vi "GoblePaths.vi"(8 "error in (no error)":errorcluster caption="错误输入（无错误）", 11 "文件名称":string) -> (0 "error out":errorcluster caption="错误输出", 2 "文件完整路径":path, 3 "文件路径":path)   [LabVIEW 2018]
panel:
  out "文件夹路径":path[](array[path])
  out "文件夹名":string[](array[string])
  out "路径输出":path
  out "Application Directory":path caption="应用程序目录"
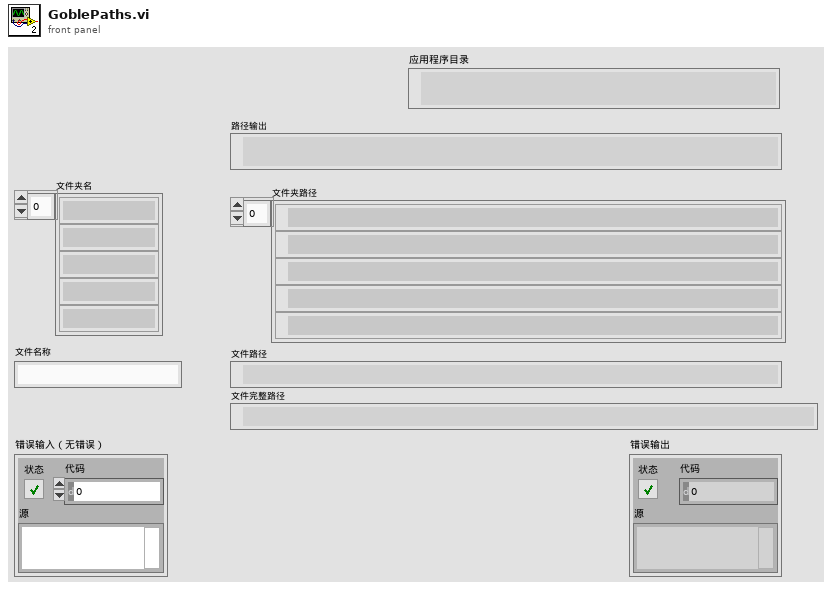
[diagram p1: front panel]
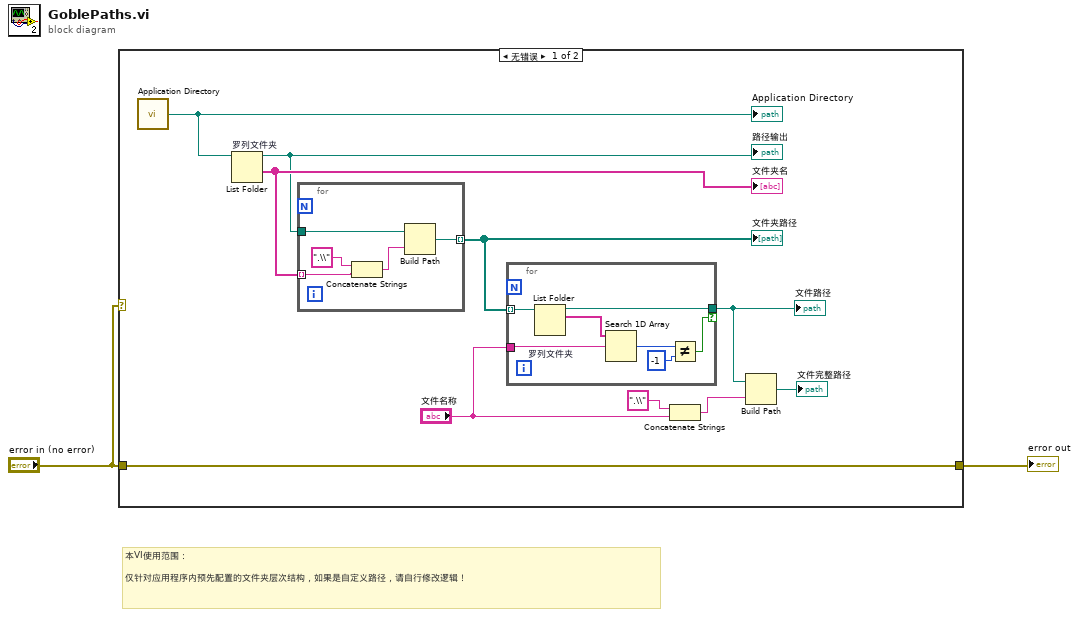
[diagram p0: block diagram]
diagram:
  # "本VI使用范围：\n\n仅针对应用程序内预先配置的文件夹层次结构，如果是自定义路径，请自行修改逻辑！"
  n1 = case shown="无错误" "error in (no error)" {
    tunnel: "error in (no error)" -> [w8 w25]
    tunnel: [w8 w25] -> w2
    frame No Error {
      n2 = call <vilib>:"Application Directory.vi"() -> ("Application Directory"=w12:path)
      "Application Directory" <- w12
      n3 = List Folder "罗列文件夹"(path=w12) -> (path out=w10:path, folder names=w11:string[])  [unwired: 3 in, 2 out]
      "路径输出" <- w10
      "文件夹名" <- w11
      n4 = for {
        tunnel: w11 -> [w22] mode=indexing
        tunnel: w10 -> [w24]
        tunnel: [w20] -> w9 mode=indexing
        n5 = Concatenate Strings(".\\" ("字符串"), w22) -> (w23:string)
        n6 = Build Path(base path=w24, name or relative path=w23) -> (appended path=w20:path)
      }
      "文件夹路径" <- w9
      n7 = for {
        tunnel: w9 -> [w19] mode=indexing
        tunnel: "文件名称" -> [w16]
        tunnel: [w18] -> w7 if=w13
        n8 = List Folder "罗列文件夹"(path=w19) -> (path out=w18:path, filenames=w17:string[])  [unwired: 3 in, 2 out]
        n9 = Search 1D Array(1D array=w17, element=w16) -> (index of element=w15:i32)  [unwired: 1 in]
        n10 = Not Equal?(x=w15, y=-1) -> (x != y?=w13:bool)
      }
      "文件路径" <- w7
      n11 = Concatenate Strings(".\\" ("字符串"), "文件名称") -> (w6:string)
      n12 = Build Path(base path=w7, name or relative path=w6) -> (appended path=→"文件完整路径":path)
    }
    frame Error {
    }
  }
  "error out" <- w2
